vi "Dynamic Event.vi"() -> ()   [LabVIEW 2020]
panel:
  in  "Trigger":bool
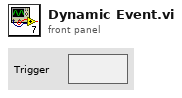
[diagram p1: front panel]
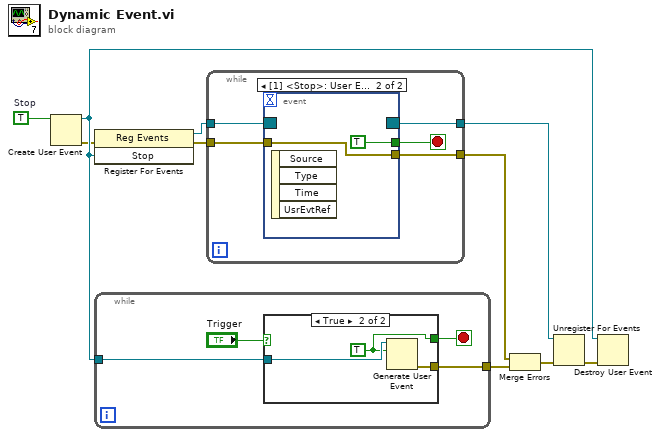
[diagram p0: block diagram]
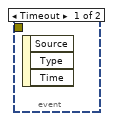
[diagram p3: hidden frame]
diagram:
  w9 = TRUE  # Stop
  n1 = Create User Event(user event datatype=w9) -> (user event=w6:refnum<user-event>, error out=w1:errorcluster)  [unwired: 1 in]
  n2 = register-events(error in=w1, w6) -> (reference out=w10:refnum<event-registration>, error out=w3:errorcluster)  [unwired: 1 in]
  n3 = while {
    tunnel: w6 -> [w14]
    tunnel: [w11] -> w5
    stop <- w12 stop-if-true
    n4 = case shown="True" "Trigger" {
      tunnel: w14 -> [_ w17]
      tunnel: [_ w16] -> w12
      tunnel: [_ w15] -> w11
      frame False {
      }
      frame True {
        w16 = TRUE
        n5 = Generate User Event(user event=w17, event data cluster=w16) -> (error out=w15:errorcluster)  [unwired: 2 in, 1 out]
      }
    }
  }
  n6 = while {
    tunnel: w10 -> [w22]
    tunnel: [w21] -> w8
    tunnel: w3 -> [w19]
    tunnel: [w18] -> w2
    stop <- w20 stop-if-true
    n7 = event shown="[1] <Stop>: User Event" {
      selector: w22 -> [_ _]
      dyn-events: [_ _] -> w21
      timeout: _ -> [_ _]
      tunnel: [_ TRUE] -> w20
      tunnel: w19 -> [_ w23]
      tunnel: [_ w23] -> w18
      event Timeout {
        n8 = event-data() -> ()  [unwired: 1 in, 3 out]
      }
      event User Event {
        n9 = event-data() -> ()  [unwired: 1 in, 4 out]
      }
    }
  }
  n10 = Merge Errors(w2, w5) -> (w4:errorcluster)
  n11 = Unregister For Events(event registration refnum=w8, error in=w4) -> (error out=w7:errorcluster)
  n12 = Destroy User Event(user event=w6, error in=w7) -> ()  [unwired: 1 out]
